vi "DAQ 디지털 버튼, 아날로그 입력 실습(강사).vi"() -> ()   [LabVIEW 2020]
uses:
  <vilib>/DAQmx/read.llb/DAQmx Read (Digital 1D Bool 1Chan 1Samp).vi
  <vilib>/DAQmx/read.llb/DAQmx Read (Analog 2D DBL NChan NSamp).vi
  <vilib>/DAQmx/create/channels.llb/DAQmx Create Channel (DI-Digital Input).vi
  <vilib>/DAQmx/create/channels.llb/DAQmx Create Channel (AI-Voltage-Basic).vi
  <vilib>/DAQmx/configure/timing.llb/DAQmx Timing (Sample Clock).vi
  <vilib>/DAQmx/miscellaneous.llb/DAQmx Fill In Error Info.vi
panel:
  out "TCM":dbl[](graph)
  out "PTM":dbl[](graph)
  in  "정지":bool
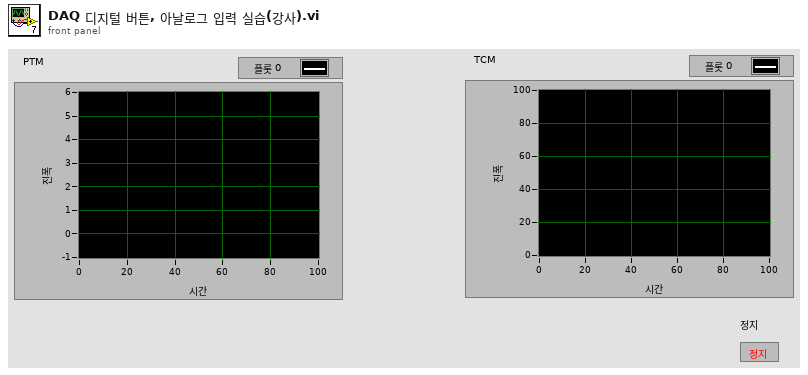
[diagram p1: front panel]
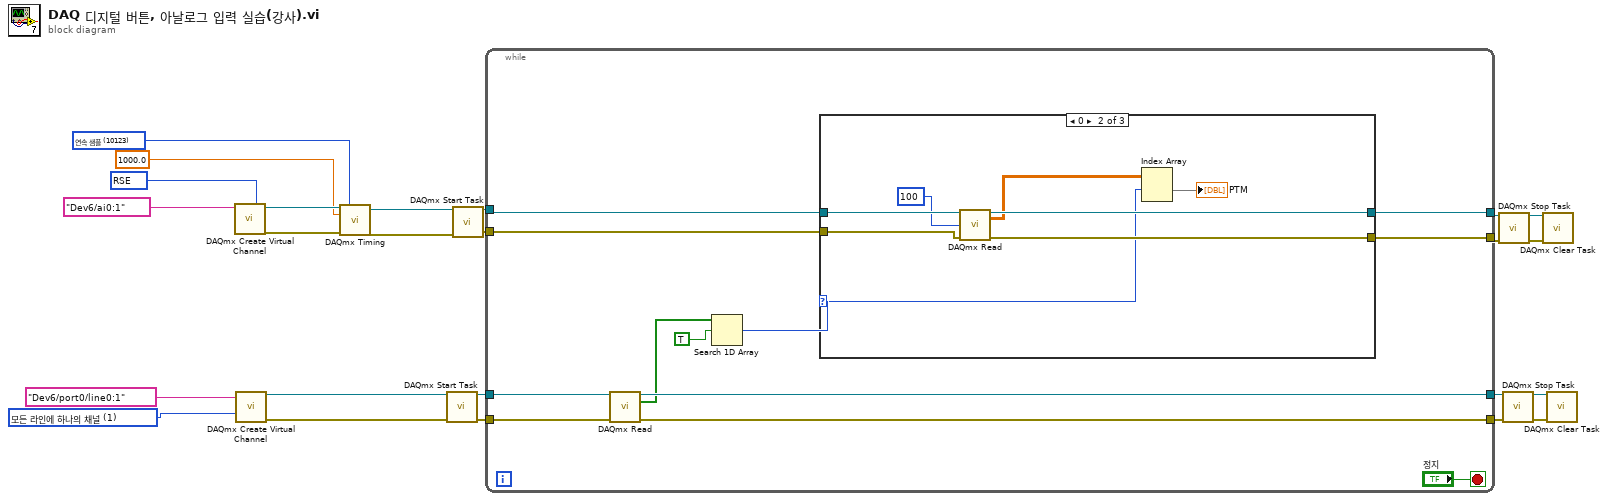
[diagram p0: block diagram]
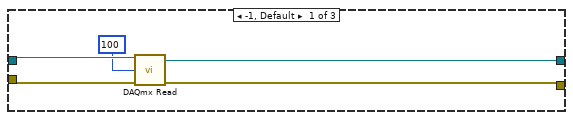
[diagram p2: hidden frame]
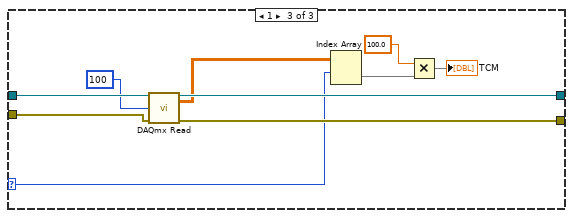
[diagram p3: hidden frame]
diagram:
  w6 = 10123 items=["유한 샘플"=10178, "연속 샘플"=10123, "하드웨어 타이밍에 의한 단일 포인트"=12522] ("sample mode")
  w7 = 10083 items=["기본"=-1, "RSE"=10083, "NRSE"=10078, "차동"=10106, "유사 차동"=12529] ("input terminal configuration")
  w17 = 1 items=["각 라인에 하나의 채널", "모든 라인에 하나의 채널"] ("line grouping")
  n1 = call-poly <vilib>:"DAQmx Create Virtual Channel.vi"("input terminal configuration"=w7, "physical channels"=tag "Dev6/ai0:1") -> ("task out"=w24:refnum<k21>, "error out"=w23:errorcluster)  [unwired: 12 in]
  n2 = call-poly <vilib>:"DAQmx Create Virtual Channel.vi"("lines"=tag "Dev6/port0/line0:1", "line grouping"=w17) -> ("task out"=w16:refnum<k21>, "error out"=w15:errorcluster)  [unwired: 12 in]
  n3 = call-poly <vilib>:"DAQmx Timing.vi"("task/channels in"=w24, "sample mode"=w6, "rate"=1000.0, "error in"=w23) -> ("task out"=w10:refnum<k21>, "error out"=w9:errorcluster)  [unwired: 10 in]
  n4 = call <vilib>:"DAQmx Start Task.vi"("task/channels in"=w16, "error in"=w15) -> ("task out"=w14:refnum<k21>, "error out"=w13:errorcluster)  [unwired: 12 in]
  n5 = call <vilib>:"DAQmx Start Task.vi"("task/channels in"=w10, "error in"=w9) -> ("task out"=w4:refnum<k21>, "error out"=w3:errorcluster)  [unwired: 12 in]
  n6 = while {
    tunnel: w14 -> [w36]
    tunnel: w13 -> [w35]
    tunnel: [w34] -> w12
    tunnel: [w33] -> w11
    tunnel: w4 -> [w32]
    tunnel: w3 -> [w31]
    tunnel: [w30] -> w2
    tunnel: [w29] -> w1
    stop <- "정지" stop-if-true
    n7 = call-poly <vilib>:"DAQmx Read.vi"("task/channels in"=w36, "error in"=w35) -> ("task out"=w34:refnum<k21>, "data"=w27:bool[], "error out"=w33:errorcluster)  [unwired: 11 in]
    n8 = Search 1D Array(1D array=w27, element=TRUE) -> (index of element=w25:i32)  [unwired: 1 in]
    n9 = case shown="0" w25 {
      selector: w25 -> [_ w43 w53]
      tunnel: w32 -> [w41 w49 w59]
      tunnel: w31 -> [w40 w48 w58]
      tunnel: [w38 w47 w57] -> w30
      tunnel: [w39 w46 w56] -> w29
      frame -1, Default {
        n10 = call-poly <vilib>:"DAQmx Read.vi"("task/channels in"=w41, "number of samples per channel"=100, "error in"=w40) -> ("task out"=w38:refnum<k21>, "error out"=w39:errorcluster)  [unwired: 10 in, 1 out]
      }
      frame 0 {
        n11 = call-poly <vilib>:"DAQmx Read.vi"("task/channels in"=w49, "number of samples per channel"=100, "error in"=w48) -> ("task out"=w47:refnum<k21>, "data"=w44:dbl[][], "error out"=w46:errorcluster)  [unwired: 10 in]
        n12 = Index Array(array=w44, index (row)=w43) -> (element=→"PTM":dbl[])  [unwired: 1 in]
      }
      frame 1 {
        n13 = call-poly <vilib>:"DAQmx Read.vi"("task/channels in"=w59, "number of samples per channel"=100, "error in"=w58) -> ("task out"=w57:refnum<k21>, "data"=w54:dbl[][], "error out"=w56:errorcluster)  [unwired: 10 in]
        n14 = Index Array(array=w54, index (row)=w53) -> (element=w52:dbl[])  [unwired: 1 in]
        n15 = Multiply(x=100.0, y=w52) -> (x*y=→"TCM":dbl[])
      }
    }
  }
  n16 = call <vilib>:"DAQmx Stop Task.vi"("task/channels in"=w2, "error in"=w1) -> ("task out"=w22:refnum<k21>, "error out"=w21:errorcluster)  [unwired: 12 in]
  n17 = call <vilib>:"DAQmx Stop Task.vi"("task/channels in"=w12, "error in"=w11) -> ("task out"=w20:refnum<k21>, "error out"=w19:errorcluster)  [unwired: 12 in]
  n18 = call <vilib>:"DAQmx Clear Task.vi"("task in"=w22, "error in"=w21) -> ()  [unwired: 13 in, 1 out]
  n19 = call <vilib>:"DAQmx Clear Task.vi"("task in"=w20, "error in"=w19) -> ()  [unwired: 13 in, 1 out]
